vi "Do.vi"(8 "error in (no error)":errorcluster, 10 "Actor in":refnum<class "Actor.lvclass">, 11 "Add Sink Msg in":refnum<class "Add Sink Msg.lvclass">) -> (0 "error out":errorcluster, 2 "Actor out":refnum<class "Actor.lvclass">)   [LabVIEW 2016, in "Event Source.lvlib" / "Add Sink Msg.lvclass"]
doc: "(<B>Filename</B>: Actor Framework.lvlib:Message.lvclass:Do.vi)\n\nDefines what a message does when it is received by an actor. Generally, a message instructs an actor to invoke one of its methods. By default, this method does nothing. A child class must override it to define behavior. Create a child class by using the Actor Framework Message Maker dialog box."
uses:
  Add Sink Msg.lvclass
  <vilib>/ActorFramework/Actor/Actor.lvclass
  Event Source/Event Source.lvclass
  C:/Program Files (x86)/National Instruments/LabVIEW 2016/vi.lib/ActorFramework/Actor/Actor.lvclass
  Add Sink Msg.lvclass/Add Sink Msg.ctl
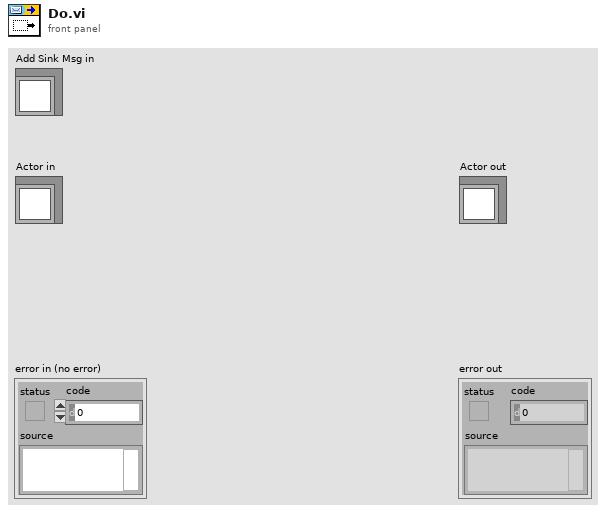
[diagram p1: front panel]
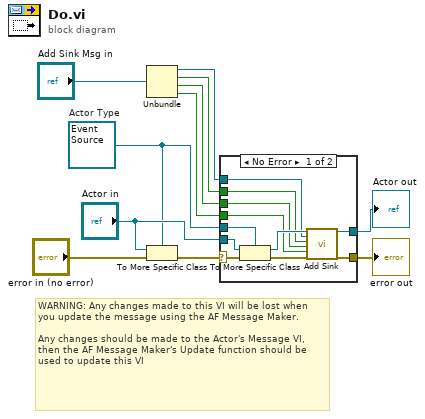
[diagram p0: block diagram]
diagram:
  w6 = refnum<class "Event Source.lvclass"> refnum  # Actor Type
  # "WARNING: Any changes made to this VI will be lost when you update the message using the AF Message Maker.\n\nAny changes should be made to the Actor's Message VI, then the AF Message Maker's Update function should be used to update this VI"
  n1 = Unbundle("Add Sink Msg in") -> (w5:refnum<class "Event Sink.lvclass">, w4:bool, w3:bool, w2:bool)
  n2 = To More Specific Class(target class=w6, reference="Actor in", error in="error in (no error)") -> (error out=w10:errorcluster)  [unwired: 1 out]
  n3 = case shown="No Error" w10 {
    selector: w10 -> [w22 w24]
    tunnel: [w17 w24] -> w9
    tunnel: [w16 w23] -> w8
    tunnel: "Actor in" -> [w21 w23]
    tunnel: w6 -> [w20 _]
    tunnel: w5 -> [w15 _]
    tunnel: w4 -> [w14 _]
    tunnel: w3 -> [w13 _]
    tunnel: w2 -> [w12 _]
    frame No Error {
      n4 = To More Specific Class ("Actor Cast")(target class=w20, reference=w21, error in=w22) -> (specific class reference=w19:refnum<class "Event Source.lvclass">, error out=w18:errorcluster)
      n5 = call "Add Sink.vi"("Event Source in"=w19, "Sink Actor"=w15, "Exclude From Broadcast (F)"=w14, "Paused (F)"=w13, "Receive Only (F)"=w12, "error in (no error)"=w18) -> ("Event Source out"=w16:refnum<class "Event Source.lvclass">, "error out"=w17:errorcluster)  [unwired: 12 in]
    }
    frame Error {
    }
  }
  "error out" <- w9
  "Actor out" <- w8
